vi "PH_Trendviewer_Powermeter.indicate Result.vi"(0 "i ref in":refnum<vi>, 5 "error in (no error)":errorcluster) -> (14 "i ref out":refnum<vi>, 19 "error out":errorcluster)   [LabVIEW 2014, in "PH_Trendviewer_Powermeter.lvlib"]
doc: "This VI displays the results"
uses:
  PH_Trendviewer_Powermeter.lvlib
  <vilib>/Analysis/NI_AALBase.lvlib
  <vilib>/Analysis/NI_AALPro.lvlib
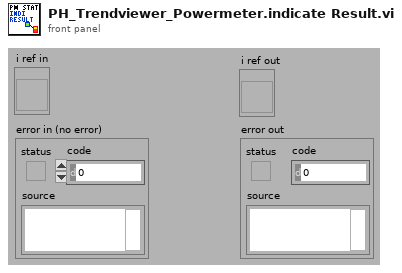
[diagram p1: front panel]
types:
  T1 = typedef "PH_Trendviewer_Powermeter.lvlib/PH_Trendviewer_Powermeter.i attribute.ctl" = cluster{"GUI Refs ":cluster{"Status":refnum<vi>, "Result Graph":refnum<vi>, "Mean Data":refnum<vi>, "Std Dev Data":refnum<vi>, "Dummy Mean":refnum<vi>, "Dummy Std Dev":refnum<vi>, "Export Data":refnum<vi>, "Stat or Trend":refnum<vi>, "Delete":refnum<vi>, "Powermeter":refnum<vi>, "Start":refnum<vi>}, "Powermeter":string, "Stat or Trend":bool, "Start":bool, "Data":cluster{"Time Stamp":timestamp, "Energy [J]":dbl}[], "Datasets strored":i32, "Dataarray Size":i32}
  T2 = cluster{"Time Stamp":timestamp, "Energy [J]":dbl}[]
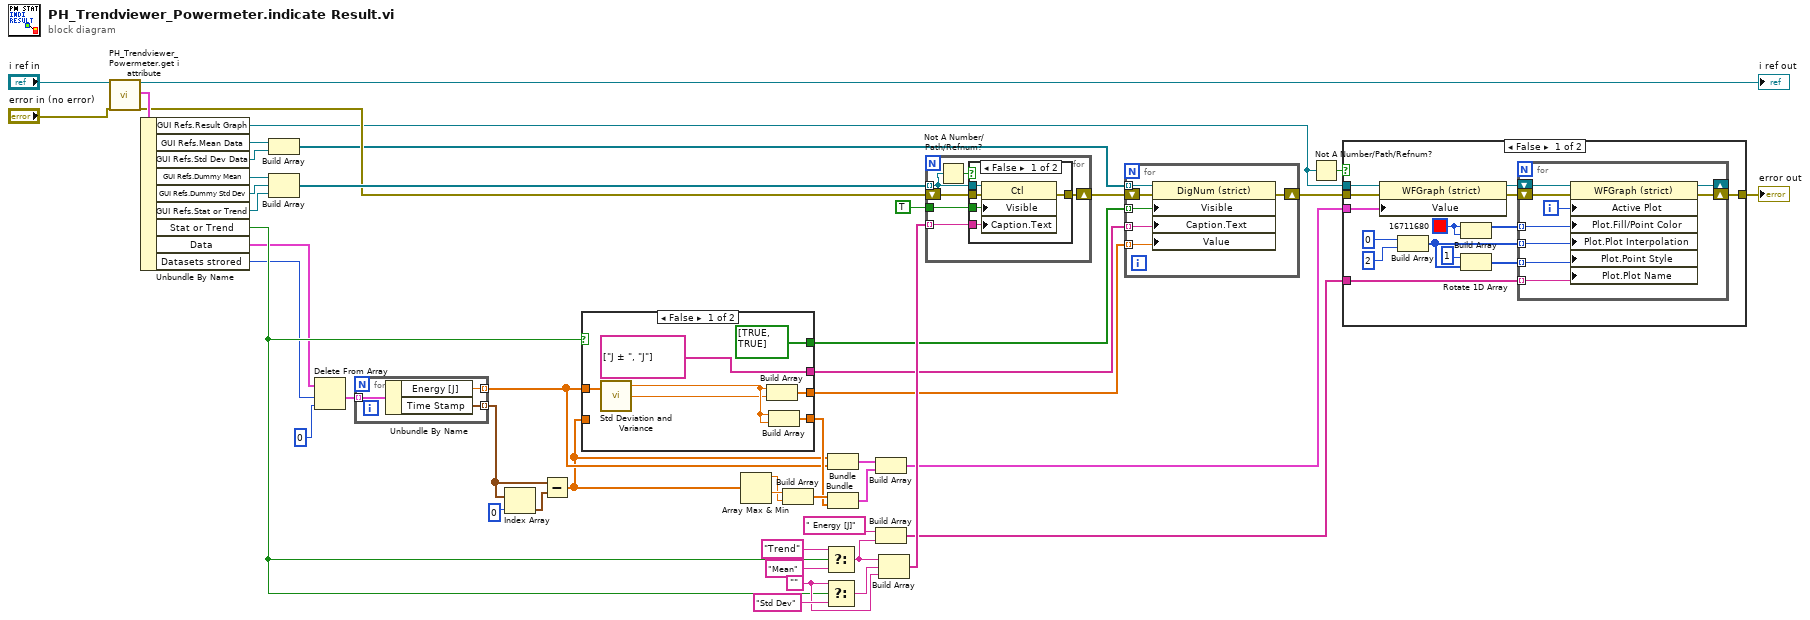
[diagram p0: block diagram]
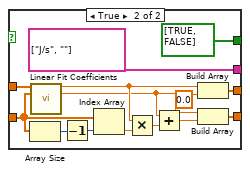
[diagram p2: hidden frame]
diagram:
  w31 = ""
  n1 = call "PH_Trendviewer_Powermeter.get i attribute.vi"("i ref in"="i ref in", "error in (no error)"="error in (no error)") -> ("i ref out"=→"i ref out":refnum<vi>, "i attribute"=w45:T1, "error out"=w25:errorcluster)  [unwired: 15 in]
  n2 = Unbundle By Name(w45) -> ("GUI Refs.Result Graph"=w24:refnum<vi>, "GUI Refs.Mean Data"=w44:refnum<vi>, "GUI Refs.Std Dev Data"=w43:refnum<vi>, "GUI Refs.Dummy Mean"=w39:refnum<vi>, "GUI Refs.Dummy Std Dev"=w22:refnum<vi>, "GUI Refs.Stat or Trend"=w37:refnum<vi>, "Stat or Trend"=w23:bool, "Data"=w4:T2, "Datasets strored"=w2:i32)
  n3 = Build Array(w44, w43) -> (w21:refnum<vi>[])
  n4 = Build Array(w39, w22, w37) -> (w42:refnum<vi>[])
  n5 = Delete From Array(array=w4, length=w2, index=0) -> (deleted portion=w5:T2)  [unwired: 1 out]
  n6 = for {
    tunnel: w5 -> [w50] mode=indexing
    tunnel: [w48] -> w12 mode=indexing
    tunnel: [w49] -> w9 mode=indexing
    n7 = Unbundle By Name(w50) -> ("Energy [J]"=w49:dbl, "Time Stamp"=w48:timestamp)
  }
  n8 = Index Array(array=w12, index=0) -> (element=w10:timestamp)
  n9 = Subtract(x=w12, y=w10) -> (x-y=w8:dbl[])
  n10 = case shown="False" w23 {
    tunnel: w9 -> [w55 w69]
    tunnel: [w57 w71] -> w18
    tunnel: [string[] ["J ± ", "J"] string[] ["J/s", ""]] -> w17
    tunnel: [bool[] [TRUE, TRUE] bool[] [TRUE, FALSE]] -> w16
    tunnel: [w56 w68] -> w15
    tunnel: w8 -> [_ w67]
    frame False {
      n11 = call <vilib>:"Std Deviation and Variance.vi"("X"=w55) -> ("mean"=w54:dbl, "standard deviation"=w53:dbl)  [unwired: 1 in, 1 out]
      n12 = Build Array(w54, w53) -> (w57:dbl[])
      n13 = Build Array(w54, w54) -> (w56:dbl[])
    }
    frame True {
      n14 = Array Size(array=w67) -> (size(s)=w66:i32)
      n15 = call <vilib>:"Linear Fit Coefficients.vi"("Y"=w69, "X"=w67) -> ("slope"=w63:dbl, "intercept"=w61:dbl)  [unwired: 11 in, 1 out]
      n16 = Decrement(x=w66) -> (x-1=w65:i32)
      n17 = Index Array(array=w67, index=w65) -> (element=w64:dbl)
      n18 = Multiply(x=w63, y=w64) -> (x*y=w62:dbl)
      n19 = Add(x=w61, y=w62) -> (x+y=w60:dbl)
      n20 = Build Array(w63, 0.0 ("element")) -> (w71:dbl[])
      n21 = Build Array(w61, w60) -> (w68:dbl[])
    }
  }
  n22 = Array Max & Min(array=w8) -> (max value=w40:dbl, min value=w41:dbl)  [unwired: 2 out]
  n23 = Build Array(w41, w40) -> (w38:dbl[])
  n24 = Select(t="Trend" ("Plot.Plot Name"), s=w23, f="Mean") -> (s? t:f=w13:string)
  n25 = Select(t=w31, s=w23, f="Std Dev") -> (s? t:f=w36:string)
  n26 = Bundle(w8, w9) -> (w20:cluster{dbl[], dbl[]})  [unwired: 1 in]
  n27 = Bundle(w38, w15) -> (w19:cluster{dbl[], dbl[]})  [unwired: 1 in]
  n28 = Build Array(w20, w19) -> (w29:cluster{dbl[], dbl[]}[])
  n29 = Build Array(" Energy [J]", w13) -> (w30:string[])
  n30 = Build Array(w13, w36, w31) -> (w32:string[])
  n31 = for {
    tunnel: w42 -> [w73] mode=indexing
    shift-right: [w76] -> w6
    shift-left: w25 -> [w77]
    tunnel: w32 -> [w75] mode=indexing
    tunnel: TRUE -> [w72]
    n32 = Not A Number/Path/Refnum?(number/path/refnum=w73) -> (NaN/Path/Refnum?=w74:bool)
    n33 = case shown="False" w74 {
      tunnel: w73 -> [w82 _]
      tunnel: w77 -> [w81 w83]
      tunnel: [w80 w83] -> w76
      tunnel: w75 -> [w79 _]
      tunnel: w72 -> [w78 _]
      frame False {
        n34 = property class="Ctl"(reference=w82, error in=w81, "Visible"=w78, "Caption.Text"=w79) -> (error out=w80:errorcluster)  [unwired: 1 out]
      }
      frame True {
      }
    }
  }
  n35 = for {
    tunnel: w21 -> [w89] mode=indexing
    tunnel: w18 -> [w88] mode=indexing
    shift-right: [w86] -> w28
    shift-left: w6 -> [w87]
    tunnel: w16 -> [w84] mode=indexing
    tunnel: w17 -> [w85] mode=indexing
    n36 = property class="DigNum (strict)"(reference=w89, error in=w87, "Visible"=w84, "Caption.Text"=w85, "Value"=w88) -> (error out=w86:errorcluster)  [unwired: 1 out]
  }
  n37 = Not A Number/Path/Refnum?(number/path/refnum=w24) -> (NaN/Path/Refnum?=w26:bool)
  n38 = case shown="False" w26 {
    tunnel: w30 -> [w96 _]
    tunnel: w29 -> [w95 _]
    tunnel: w24 -> [w94 _]
    tunnel: w28 -> [w92 w113]
    tunnel: [w90 w113] -> w27
    frame False {
      w103 = u32 16711680 ("Color Box")
      n39 = property class="WFGraph (strict)"(reference=w94, error in=w92, "Value"=w95) -> (reference out=w93:refnum<vi>, error out=w91:errorcluster)
      n40 = Build Array(u8 0 ("Plot.Plot Interpolation"), u8 2 ("Plot.Plot Interpolation")) -> (w99:u8[])
      n41 = Build Array(w103, w103) -> (w102:u32[])
      n42 = Rotate 1D Array(1:w99, 2:1 ("n")) -> (0:w97:u8[])
      n43 = for {
        shift-right: [w112] -> _
        shift-left: w93 -> [w111]
        shift-right: [w110] -> w90
        shift-left: w91 -> [w109]
        tunnel: w102 -> [w107] mode=indexing
        tunnel: w99 -> [w106] mode=indexing
        tunnel: w97 -> [w105] mode=indexing
        tunnel: w96 -> [w104] mode=indexing
        i -> [w108]
        n44 = property class="WFGraph (strict)"(reference=w111, error in=w109, "Active Plot"=w108, "Plot.Fill/Point Color"=w107, "Plot.Plot Interpolation"=w106, "Plot.Point Style"=w105, "Plot.Plot Name"=w104) -> (reference out=w112:refnum<vi>, error out=w110:errorcluster)
      }
    }
    frame True {
    }
  }
  "error out" <- w27
